vi "Get Descendants.vi"(8 "error in (no error)":errorcluster, 11 "TreeNode in":refnum<class "TreeNode.lvclass">) -> (0 "error out":errorcluster, 1 "TreeNodeArray":refnum<class "TreeNode.lvclass">[](array[class]), 2 "Descendants":i64[](array[numeric]), 3 "TreeNode out":refnum<class "TreeNode.lvclass">)   [LabVIEW 2012, in "MDSplus.lvlib" / "TreeNode.lvclass"]
uses:
  <vilib>/MDSplus/Classes/Data_Class/TreeNode_Class/TreeNode.lvclass
  MDSobjectsLVShr.dll
  <vilib>/MDSplus/Classes/Data_Class/Data.lvclass
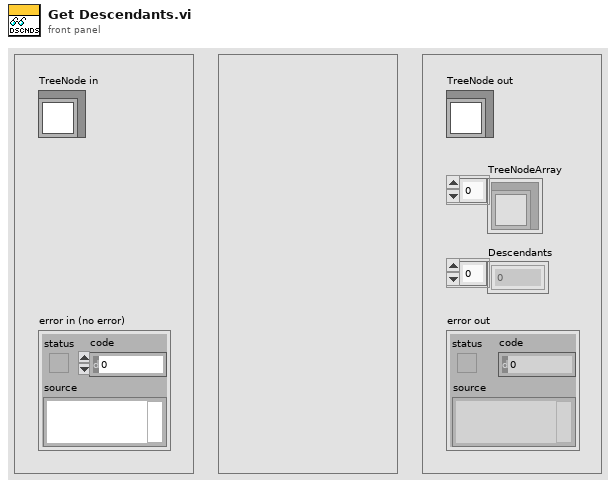
[diagram p1: front panel]
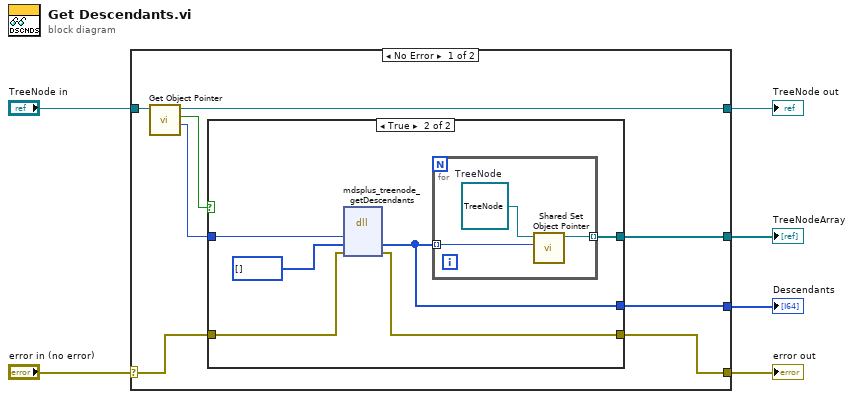
[diagram p0: block diagram]
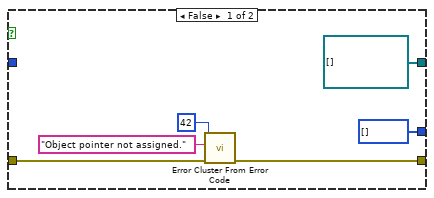
[diagram p2: hidden frame]
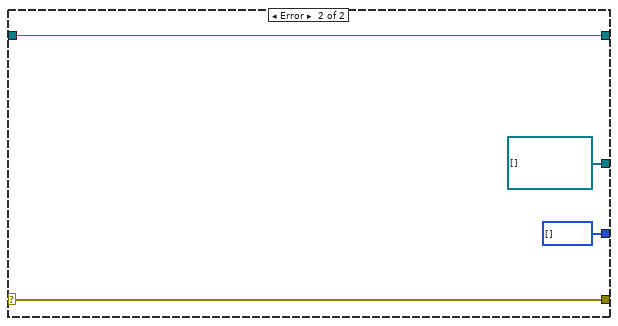
[diagram p3: hidden frame]
diagram:
  n1 = case shown="No Error" "error in (no error)" {
    selector: "error in (no error)" -> [w11 w33]
    tunnel: [w10 w33] -> w5
    tunnel: [w9 w32] -> w3
    tunnel: "TreeNode in" -> [w12 w32]
    tunnel: [w8 i64[] [] ("PtrArrayHdlOut")] -> w2
    tunnel: [w7 refnum<class "TreeNode.lvclass">[] []] -> w1
    frame No Error {
      n2 = call-dynamic "Get Object Pointer.vi"("Data in"=w12) -> ("Object Pointer"=w13:i64, "Assigned object pointer?"=w14:bool, "Data out"=w9:refnum<class "TreeNode.lvclass">)  [unwired: 8 in]
      n3 = case shown="True" w14 {
        tunnel: w13 -> [_ w26]
        tunnel: w11 -> [w18 w25]
        tunnel: [w17 w24] -> w10
        tunnel: [i64[] [] ("PtrArrayHdlOut") w22] -> w8
        tunnel: [refnum<class "TreeNode.lvclass">[] [] w21] -> w7
        frame False {
          n4 = call <vilib>:"Error Cluster From Error Code.vi"("error in (no error)"=w18, "error message (\"\")"="Object pointer not assigned." ("error message (\"\")"), "error code (0)"=42) -> ("error out"=w17:errorcluster)  [unwired: 6 in]
        }
        frame True {
          n5 = dll-call lib="MDSobjectsLVShr.dll" fn="mdsplus_treenode_getDescendants"("lvTreeNodePtr"=w26, "PtrArrayHdlOut"=i64[] [], "error"=w25) -> ("PtrArrayHdlOut"=w22:i64[], "error"=w24:errorcluster)  [unwired: 5 in, 2 out]
          n6 = for {
            tunnel: w22 -> [w27] mode=indexing
            tunnel: [w28] -> w21 mode=indexing
            w29 = refnum<class "TreeNode.lvclass"> refnum  # TreeNode
            n7 = call <vilib>:"Shared Set Object Pointer.vi"("Object Pointer"=w27, "Data in"=w29) -> ("Data out"=w28:refnum<class "TreeNode.lvclass">)  [unwired: 9 in]
          }
        }
      }
    }
    frame Error {
    }
  }
  "error out" <- w5
  "TreeNode out" <- w3
  "Descendants" <- w2
  "TreeNodeArray" <- w1
